vi "Format Variant Into String__ogtk.vi"(0 "Input String":string, 2 "Format String":string, 7 "error in (no error)":errorcluster, 11 "Variant":variant) -> (4 "Output String":string, 8 "error out":errorcluster)   [LabVIEW 2018]
doc: "Overcomes a limitation of \"Format Into String\" by allowing variant data types to be used. This VI supports variant data for all LabVIEW data types supported by \"Format Into String\". \n\n<b>Notes:</b>\n<b>Format string</b> input may optionally be passed as a variant attribute named \"Format String\".\n<b>ISO 8601</b> is used as the default formating for Timestamp unless otherwise specified. <b>Timestamp</b> data must use the <b>Format String:</b> %T (or variations of %T), otherwise it will return an error."
panel:
  # "Please visit http://www.OpenG.org to learn about the\nOpen Source LabVIEW software movement.\n\nNOTICE -- YOU MUST LEAVE THIS NOTICE IN PLACE.  PER THE TERMS OF THE LICENSE BELOW, YOU MAY SUBLICENSE THIS SOFTWARE \nIN ANY WAY THAT DOES NOT CONFLICT WITH THIS LICENSE.\n\n### BSD License (http://www.opensource.org/licenses/bsd-license.php) Begin ###\n \nCopyright (c) 2002-2004, Jim Kring <jim@jimkring.com>\nCopyright (c) 2004, Michael C. Ashe <michael.ashe@imaginatics.com>\nCopyright (c) 2011, Jonathon Green <jg@jgcode.net>\nCopyright (c) 2011, Phillip Brooks <pbrooks100@gmail.com>\nCopyright (c) 2011, Jonas Mellroth<jonas.mellroth@wireflow.se>\n\nAll rights reserved.\n\nRedistribution and use in source and binary forms, with or without modification, are permitted provided that the following conditions are met:\n\n    * Redistributions of source code must retain the above copyright notice, this list of conditions and the following disclaimer.\n    * Redistributions in binary form must reproduce the above copyright notice, this list of conditions and the following disclaimer in the \n       documentation and/or other materials provided with the distribution.\n    * Neither the name of SciWare, James Kring, Inc., nor the names of its contributors may be used to endorse or promote products derived \n       from this software without specific prior written permission.\n\nTHIS SOFTWARE IS PROVIDED BY THE COPYRIGHT HOLDERS AND CONTRIBUTORS \"AS IS\" AND ANY EXPRESS OR IMPLIED WARRANTIES, \nINCLUDING, BUT NOT LIMITED TO, THE IMPLIED WARRANTIES OF MERCHANTABILITY AND FITNESS FOR A PARTICULAR PURPOSE ARE \nDISCLAIMED. IN NO EVENT SHALL THE COPYRIGHT OWNER OR CONTRIBUTORS BE LIABLE FOR ANY DIRECT, INDIRECT, INCIDENTAL,\n SPECIAL, EXEMPLARY, OR CONSEQUENTIAL DAMAGES (INCLUDING, BUT NOT LIMITED TO, PROCUREMENT OF SUBSTITUTE GOODS OR \nSERVICES; LOSS OF USE, DATA, OR PROFITS; OR BUSINESS INTERRUPTION) HOWEVER CAUSED AND ON ANY THEORY OF LIABILITY, \nWHETHER IN CONTRACT, STRICT LIABILITY, OR TORT (INCLUDING NEGLIGENCE OR OTHERWISE) ARISING IN ANY WAY OUT OF THE USE \nOF THIS SOFTWARE, EVEN IF ADVISED OF THE POSSIBILITY OF SUCH DAMAGE.\n\n### BSD License End ###"
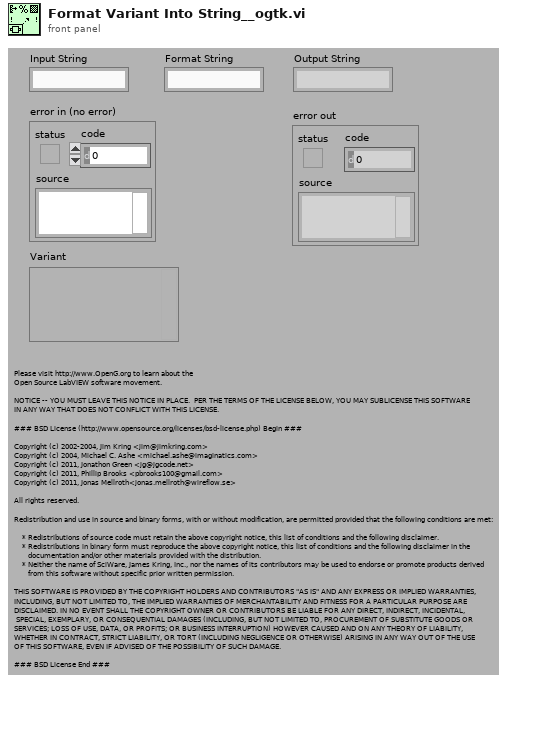
[diagram p1: front panel]
types:
  T1 = typedef "Type Descriptor Enumeration__ogtk.ctl" = enum8{"<Null>", "I8", "I16", "I32", "I64", "U8", "U16", "U32", "U64", "SGL", "DBL", "EXT", "CSG", "CDB", "CXT", "0x0F", "0x10", "0x11", "0x12", "0x13", "0x14", "Enum U8", "Enum U16", "Enum U32", "Enum U64", "SGL PQ", "DBL PQ", "EXT PQ", "CSG PQ", "CDB PQ", "CXT PQ", "0x1F", "0x20", "Boolean", "0x22", "0x23", "0x24", "0x25", "0x26", "0x27", "0x28", "0x29", "0x2A", "0x2B", "0x2C", "0x2D", "0x2E", "0x2F", "String", "0x31", "Path", "Pict", "0x34", "0x35", "0x36", "DAQ", "0x38", "0x39", "0x3A", "0x3B", "0x3C", "0x3D", "0x3E", "0x3F", "Array", "0x41", "0x42", "0x43", "0x44", "0x45", "0x46", "0x47", "0x48", "0x49", "0x4A", "0x4B", "0x4C", "0x4D", "0x4E", "0x4F", "Cluster", "0x51", "0x52", "Variant", "Waveform", "0x55", "0x56", "0x57", "0x58", "0x59", "0x5A", "0x5B", "0x5C", "0x5D", "0x5E", "0x5F", "0x60", "0x61", "0x62", "0x63", "0x64", "0x65", "0x66", "0x67", "0x68", "0x69", "0x6A", "0x6B", "0x6C", "0x6D", "0x6E", "0x6F", "Refnum"}
  T2 = typedef "Refnum Subtype Enum__ogtk.ctl" = enum8{"Generic", "Datalog File Refnum", "Byte Stream File Refnum", "Device Refnum", "Occurence Refnum", "TCP Connection Refnum", "VISA Refnum (Obsolete)", "Automation Renum", "VI Server Refnum", "Menu Refnum", "IVI Refnum (Obsolete)", "IMAQ Session", "0x0C", "Datasocket Refnum", "VISA Resource", "IVI Logical Name", "UDP Connection Refnum", "Notifier Refnum", "Queue Refnum", "IrDA Refnum", "Hardware Plugin Refnum", "Hardware Plugin Tag Refnum", "DAQmx Refnum", "Event Registration Refnum", ".NET Refnum", "User Event Refnum", "0x1A", "Event Callback", "0x1C", "0x1D", "Only Used Internal to LabVIEW", "Bluetooth", "Data Value References", "RT FIFO", "TDM Streaming"}
  T3 = typedef "Waveform Subtype Enum__ogtk.ctl" = enum8{"<Not a Waveform Type>", "0x01", "Analog 16-bit signed", "Analog Double-Precision", "0x04", "Analog Single Precision", "Timestamp", "Digital Data", "Digital Waveform", "Dynamic Data", "Analog Extended-Precision", "Analog 8-bit unsigned", "Analog 16-bit unsigned", "Analog 32-bit unsigned", "Analog 8-bit signed", "Analog 32-bit signed", "Analog Complex Single-Precision", "Analog Complex Double-Precision", "Analog Complex Extended Precision", "Analog 64-bit signed", "Analog 64-bit unsigned"}
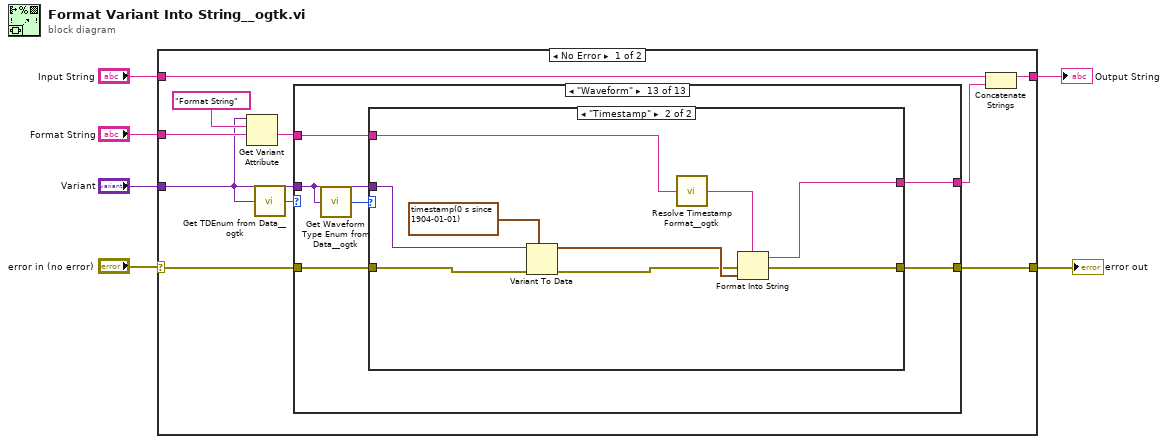
[diagram p0: block diagram]
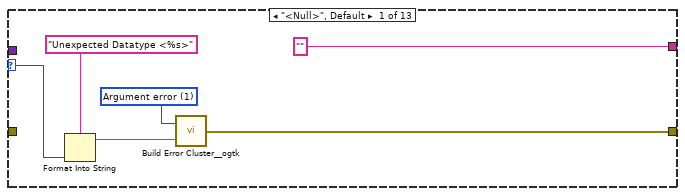
[diagram p2: hidden frame]
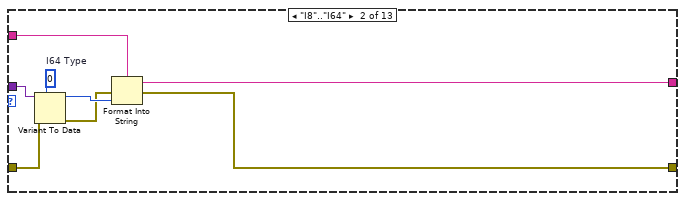
[diagram p3: hidden frame]
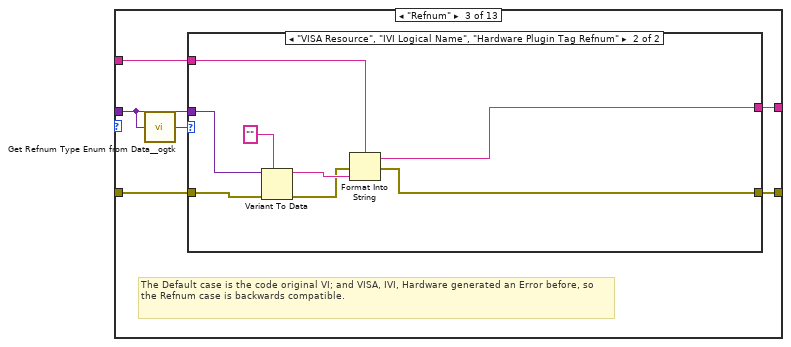
[diagram p4: hidden frame]
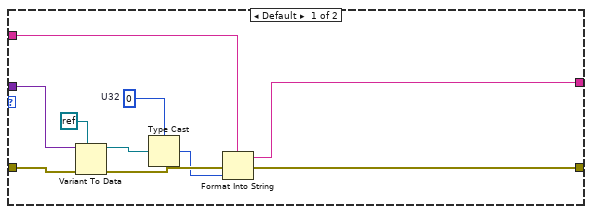
[diagram p5: hidden frame]
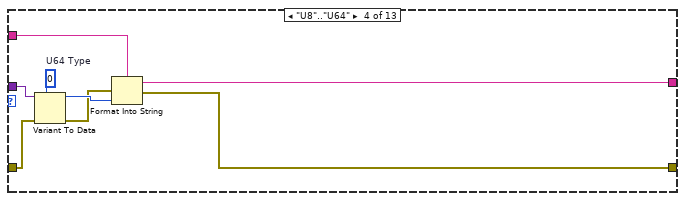
[diagram p6: hidden frame]
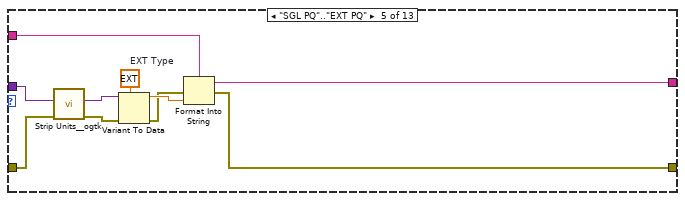
[diagram p7: hidden frame]
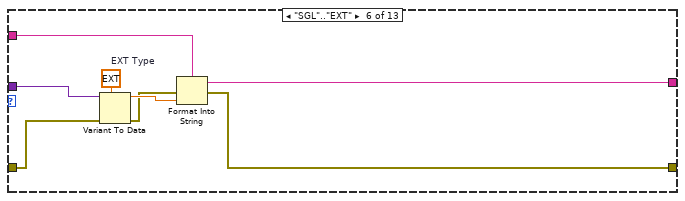
[diagram p8: hidden frame]
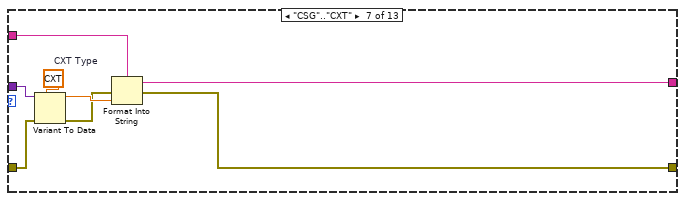
[diagram p9: hidden frame]
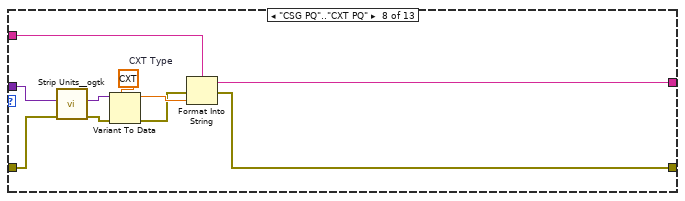
[diagram p10: hidden frame]
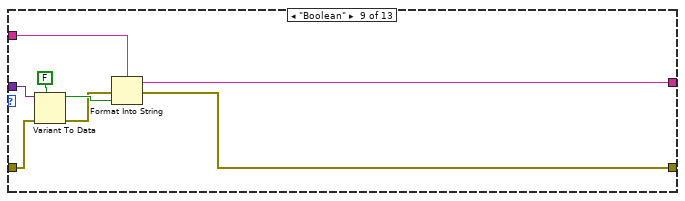
[diagram p11: hidden frame]
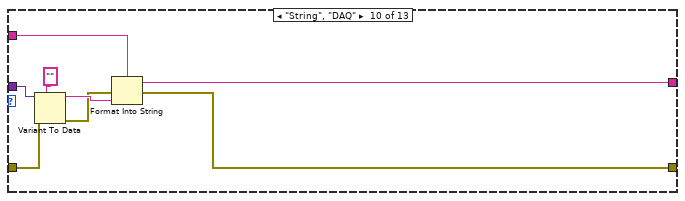
[diagram p12: hidden frame]
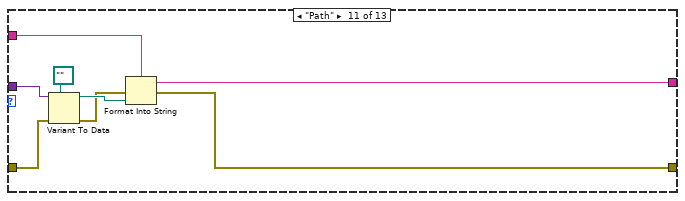
[diagram p13: hidden frame]
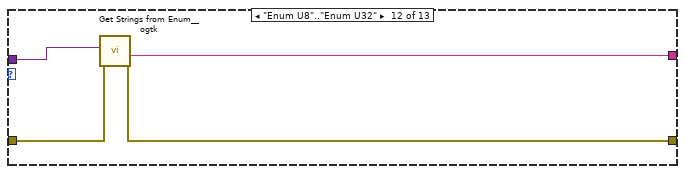
[diagram p14: hidden frame]
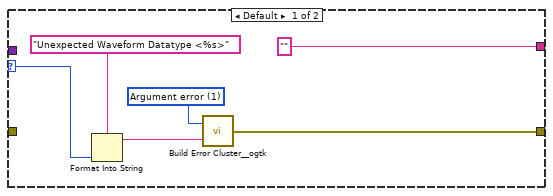
[diagram p15: hidden frame]
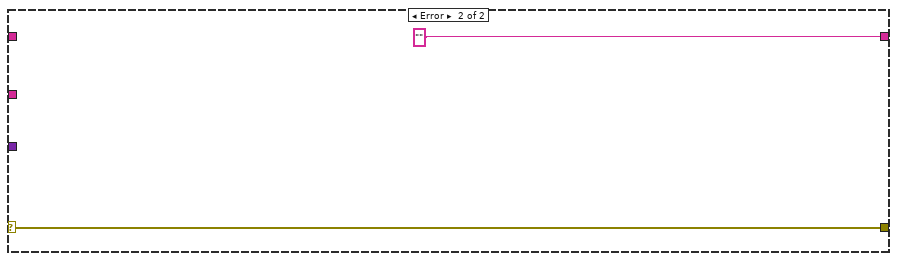
[diagram p16: hidden frame]
diagram:
  n1 = case shown="No Error" "error in (no error)" {
    selector: "error in (no error)" -> [w14 w149]
    tunnel: "Input String" -> [w11 _]
    tunnel: [w15 ""] -> w5
    tunnel: "Format String" -> [w10 _]
    tunnel: "Variant" -> [w8 _]
    tunnel: [w13 w149] -> w1
    frame No Error {
      n2 = Get Variant Attribute(Variant=w8, name="Format String", default value (empty Variant)=w10) -> (value=w9:string)  [unwired: 1 in, 3 out]
      n3 = call <userlib>:"Get TDEnum from Data__ogtk.vi"("Data"=w8) -> ("Type Descriptor Enumeration"=w7:T1)  [unwired: 4 in]
      n4 = case shown="\"Waveform\"" w7 {
        selector: w7 -> [w18 _ _ _ _ _ _ _ _ _ _ _ _]
        tunnel: w8 -> [_ w29 w32 w61 w65 w74 w87 w91 w106 w114 w122 w126 w131]
        tunnel: w9 -> [_ w27 w31 w59 w70 w78 w85 w96 w99 w112 w120 _ w127]
        tunnel: ["" w26 w33 w58 w69 w77 w84 w95 w104 w111 w119 w124 w128] -> w16
        tunnel: [w17 w23 w34 w55 w67 w75 w81 w93 w100 w108 w115 w123 w129] -> w13
        tunnel: w14 -> [_ w25 w35 w57 w64 w73 w83 w90 w102 w107 w117 w125 w130]
        frame "<Null>", Default {
          w21 = 1 items=["No error", "Argument error", "Memory is full", "Out of zone", "End of file", "File already open", "Generic file I/O error", "File not found", "File permission error", "Disk is full", "Duplicate path", "Too many files open", "System feature not enabled", "Resource file not found", "Cannot add resource", "Resource not found", "Image not found", "Image memory error", "Pen does not exist", "Config type invalid", "Config token not found", "Config parse error", "Config memory error", "Bad external code format", "Bad external code offset", "External code not present", "Null window", "Destroy window error", "Null menu", "Print aborted", "Bad print record", "Print driver error", "Windows error during printing", "Memory error during printing", "Print dialog error", "Generic print error", "Invalid device refnum", "Device not found", "Device parameter error", "Device unit error", "Cannot open device", "Device call aborted", "Generic error", "Cancelled by user", "Object ID too low", "Object ID too high", "Object not in heap", "Unknown heap", "Unknown object (invalid DefProc)", "Unknown object (DefProc not in table)", "Message out of range", "Invalid (null) method", "Unknown message", "Manager call not supported", "Bad address", "Network operation in progress", "Network operation timed out", "Connection is busy", "Network attribute not supported", "Network error", "Address in use", "System out of memory", "Connection aborted", "Connection refused", "Not connected", "Already connected", "Connection closed", "Initialization error (interapplication manager)", "Bad occurrence", "Wait on unbound occurrence handler", "Occurrence queue overflow", "Datalog type conflict", "Unused", "Unrecognized type (interapplication manager)", "Memory corrupt", "Failed to make temporary DLL", "Old CIN version", "Drag socket not found", "Failed to load drop-object", "Failed to register OLE object", "Failed to release OLE object", "Format specifier type mismatch", "Unknown format specifier", "Too few format specifiers", "Too many format specifiers", "Scan failed", "Newer CIN version", "Error converting to variant", "Runtime menu error", "Password tampered", "Variant attribute not found", "Incompatible variant data type", "Event data is not available", "Event Store is not present", "Occurrence is not found", "Event Queue is not created", "Event info is not available", "Refnum passed is NULL", "Error retrieving Class GUID", "Error retrieving CoClass GUID", "Error retrieving TypeLib GUID.", "Bad built application magic bytes.", "Specific driver is different from the specific driver associated with the Logical Name.", "There is no session opened to the class driver.", "Max Error", "MAX - Error with config objects", "MAX - Error loading configuration", "MAX - Group not supported"]
          n5 = Format Into String(format string="Unexpected Datatype <%s>" ("Format String"), w18) -> (resulting string=w19:string)  [unwired: 2 in, 1 out]
          n6 = call <userlib>:"Build Error Cluster__ogtk.vi"("String to Prepend to source (\"\")"=w19, "code"=w21) -> ("error out"=w17:errorcluster)
        }
        frame "I8".."I64" {
          w30 = i64 0  # I64 Type
          n7 = Variant To Data(error in=w25, type=w30, Variant=w29) -> (data=w28:i64, error out=w24:errorcluster)
          n8 = Format Into String(format string=w27, error in=w24, w28) -> (resulting string=w26:string, error out=w23:errorcluster)  [unwired: 1 in]
        }
        frame "Refnum" {
          # "The Default case is the code original VI; and VISA, IVI, Hardware generated an Error before, so the Refnum case is backwards compatible."
          n9 = call <userlib>:"Get Refnum Type Enum from Data__ogtk.vi"("Data"=w32) -> ("Refnum Subtype Enum"=w36:T2)  [unwired: 4 in]
          n10 = case shown="\"VISA Resource\", \"IVI Logical Name\", \"Hardware Plugin Tag Refnum\"" w36 {
            tunnel: w35 -> [w46 w51]
            tunnel: [w37 w47] -> w34
            tunnel: [w38 w50] -> w33
            tunnel: w32 -> [w45 w48]
            tunnel: w31 -> [w39 w49]
            frame Default {
              w42 = u32 0  # U32
              n11 = Variant To Data(error in=w46, type=refnum<k0> refnum, Variant=w45) -> (data=w43:refnum<k0>, error out=w41:errorcluster)
              n12 = Type Cast(type=w42, x=w43) -> (*(type *) &x=w40:u32)
              n13 = Format Into String(format string=w39, error in=w41, w40) -> (resulting string=w38:string, error out=w37:errorcluster)  [unwired: 1 in]
            }
            frame "VISA Resource", "IVI Logical Name", "Hardware Plugin Tag Refnum" {
              n14 = Variant To Data(error in=w51, type="" ("String Value"), Variant=w48) -> (data=w54:string, error out=w53:errorcluster)
              n15 = Format Into String(format string=w49, error in=w53, w54) -> (resulting string=w50:string, error out=w47:errorcluster)  [unwired: 1 in]
            }
          }
        }
        frame "U8".."U64" {
          w62 = u64 0  # U64 Type
          n16 = Variant To Data(error in=w57, type=w62, Variant=w61) -> (data=w60:u64, error out=w56:errorcluster)
          n17 = Format Into String(format string=w59, error in=w56, w60) -> (resulting string=w58:string, error out=w55:errorcluster)  [unwired: 1 in]
        }
        frame "SGL PQ".."EXT PQ" {
          w72 = ext 0.0  # EXT Type
          n18 = call <userlib>:"Strip Units__ogtk.vi"("error in (no error)"=w64, "Number or 1D array with units"=w65) -> ("error out"=w63:errorcluster, "Pure Number(s) (base units)"=w66:variant)  [unwired: 8 in]
          n19 = Variant To Data(error in=w63, type=w72, Variant=w66) -> (data=w71:ext, error out=w68:errorcluster)
          n20 = Format Into String(format string=w70, error in=w68, w71) -> (resulting string=w69:string, error out=w67:errorcluster)  [unwired: 1 in]
        }
        frame "SGL".."EXT" {
          w80 = ext 0.0  # EXT Type
          n21 = Variant To Data(error in=w73, type=w80, Variant=w74) -> (data=w79:ext, error out=w76:errorcluster)
          n22 = Format Into String(format string=w78, error in=w76, w79) -> (resulting string=w77:string, error out=w75:errorcluster)  [unwired: 1 in]
        }
        frame "CSG".."CXT" {
          w88 = cxt 0.0+0.0i  # CXT Type
          n23 = Variant To Data(error in=w83, type=w88, Variant=w87) -> (data=w86:cxt, error out=w82:errorcluster)
          n24 = Format Into String(format string=w85, error in=w82, w86) -> (resulting string=w84:string, error out=w81:errorcluster)  [unwired: 1 in]
        }
        frame "CSG PQ".."CXT PQ" {
          w98 = cxt 0.0+0.0i  # CXT Type
          n25 = call <userlib>:"Strip Units__ogtk.vi"("error in (no error)"=w90, "Number or 1D array with units"=w91) -> ("error out"=w89:errorcluster, "Pure Number(s) (base units)"=w92:variant)  [unwired: 8 in]
          n26 = Variant To Data(error in=w89, type=w98, Variant=w92) -> (data=w97:cxt, error out=w94:errorcluster)
          n27 = Format Into String(format string=w96, error in=w94, w97) -> (resulting string=w95:string, error out=w93:errorcluster)  [unwired: 1 in]
        }
        frame "Boolean" {
          n28 = Variant To Data(error in=w102, type=FALSE, Variant=w106) -> (data=w105:bool, error out=w101:errorcluster)
          n29 = Format Into String(format string=w99, error in=w101, w105) -> (resulting string=w104:string, error out=w100:errorcluster)  [unwired: 1 in]
        }
        frame "String", "DAQ" {
          n30 = Variant To Data(error in=w107, type="", Variant=w114) -> (data=w113:string, error out=w109:errorcluster)
          n31 = Format Into String(format string=w112, error in=w109, w113) -> (resulting string=w111:string, error out=w108:errorcluster)  [unwired: 1 in]
        }
        frame "Path" {
          n32 = Variant To Data(error in=w117, type=path "", Variant=w122) -> (data=w121:path, error out=w116:errorcluster)
          n33 = Format Into String(format string=w120, error in=w116, w121) -> (resulting string=w119:string, error out=w115:errorcluster)  [unwired: 1 in]
        }
        frame "Enum U8".."Enum U32" {
          n34 = call <userlib>:"Get Strings from Enum__ogtk.vi"("error in (no error)"=w125, "Enum"=w126) -> ("error out"=w123:errorcluster, "String Value"=w124:string)  [unwired: 6 in, 2 out]
        }
        frame "Waveform" {
          n35 = call <userlib>:"Get Waveform Type Enum from Data__ogtk.vi"("Data"=w131) -> ("Waveform Subtype Enum"=w132:T3)  [unwired: 4 in]
          n36 = case shown="\"Timestamp\"" w132 {
            selector: w132 -> [w134 _]
            tunnel: w131 -> [_ w145]
            tunnel: w130 -> [_ w146]
            tunnel: [w135 w141] -> w129
            tunnel: ["" w143] -> w128
            tunnel: w127 -> [_ w140]
            frame Default {
              w138 = 1 items=["No error", "Argument error", "Memory is full", "Out of zone", "End of file", "File already open", "Generic file I/O error", "File not found", "File permission error", "Disk is full", "Duplicate path", "Too many files open", "System feature not enabled", "Resource file not found", "Cannot add resource", "Resource not found", "Image not found", "Image memory error", "Pen does not exist", "Config type invalid", "Config token not found", "Config parse error", "Config memory error", "Bad external code format", "Bad external code offset", "External code not present", "Null window", "Destroy window error", "Null menu", "Print aborted", "Bad print record", "Print driver error", "Windows error during printing", "Memory error during printing", "Print dialog error", "Generic print error", "Invalid device refnum", "Device not found", "Device parameter error", "Device unit error", "Cannot open device", "Device call aborted", "Generic error", "Cancelled by user", "Object ID too low", "Object ID too high", "Object not in heap", "Unknown heap", "Unknown object (invalid DefProc)", "Unknown object (DefProc not in table)", "Message out of range", "Invalid (null) method", "Unknown message", "Manager call not supported", "Bad address", "Network operation in progress", "Network operation timed out", "Connection is busy", "Network attribute not supported", "Network error", "Address in use", "System out of memory", "Connection aborted", "Connection refused", "Not connected", "Already connected", "Connection closed", "Initialization error (interapplication manager)", "Bad occurrence", "Wait on unbound occurrence handler", "Occurrence queue overflow", "Datalog type conflict", "Unused", "Unrecognized type (interapplication manager)", "Memory corrupt", "Failed to make temporary DLL", "Old CIN version", "Drag socket not found", "Failed to load drop-object", "Failed to register OLE object", "Failed to release OLE object", "Format specifier type mismatch", "Unknown format specifier", "Too few format specifiers", "Too many format specifiers", "Scan failed", "Newer CIN version", "Error converting to variant", "Runtime menu error", "Password tampered", "Variant attribute not found", "Incompatible variant data type", "Event data is not available", "Event Store is not present", "Occurrence is not found", "Event Queue is not created", "Event info is not available", "Refnum passed is NULL", "Error retrieving Class GUID", "Error retrieving CoClass GUID", "Error retrieving TypeLib GUID.", "Bad built application magic bytes.", "Specific driver is different from the specific driver associated with the Logical Name.", "There is no session opened to the class driver.", "Max Error", "MAX - Error with config objects", "MAX - Error loading configuration", "MAX - Group not supported"]
              n37 = Format Into String(format string="Unexpected Waveform Datatype <%s>" ("Format String"), w134) -> (resulting string=w136:string)  [unwired: 2 in, 1 out]
              n38 = call <userlib>:"Build Error Cluster__ogtk.vi"("String to Prepend to source (\"\")"=w136, "code"=w138) -> ("error out"=w135:errorcluster)
            }
            frame "Timestamp" {
              n39 = Variant To Data(error in=w146, type=timestamp(0 s since 1904-01-01) ("Time Stamp"), Variant=w145) -> (data=w144:timestamp, error out=w142:errorcluster)
              n40 = call <userlib>:"Resolve Timestamp Format__ogtk.vi"("Timestamp Format In"=w140) -> ("Timestamp Format Out"=w139:string)
              n41 = Format Into String(format string=w139, error in=w142, w144) -> (resulting string=w143:string, error out=w141:errorcluster)  [unwired: 1 in]
            }
          }
        }
      }
      n42 = Concatenate Strings(w11, w16) -> (w15:string)
    }
    frame Error {
    }
  }
  "Output String" <- w5
  "error out" <- w1
